vi "RotateToAngle.vi"(7 "X":dbl, 9 "Y":dbl, 11 "Z":dbl) -> ()   [LabVIEW 2017]
uses:
  <vilib>/Rock Robotics/WPI/ThirdParty/Phoenix-LabVIEW/Motor Controller/Controls/CTRE_Phoenix_MotorControl_ControlMode.ctl
  <vilib>/addons/control/pid/pid.llb/PID (DBL).vi
  <vilib>/addons/control/pid/NI_PID_pid.lvlib
panel:
  in  "Yaw":dbl
  in  "Rot. Point Y":dbl
  in  "Rot. Point X":dbl
  in  "Inputs":dbl[](array[numeric])
  out "Speed":dbl
  out "PID Values":cluster{"P":dbl, "I":dbl, "D":dbl}
  out "Motor Output":dbl
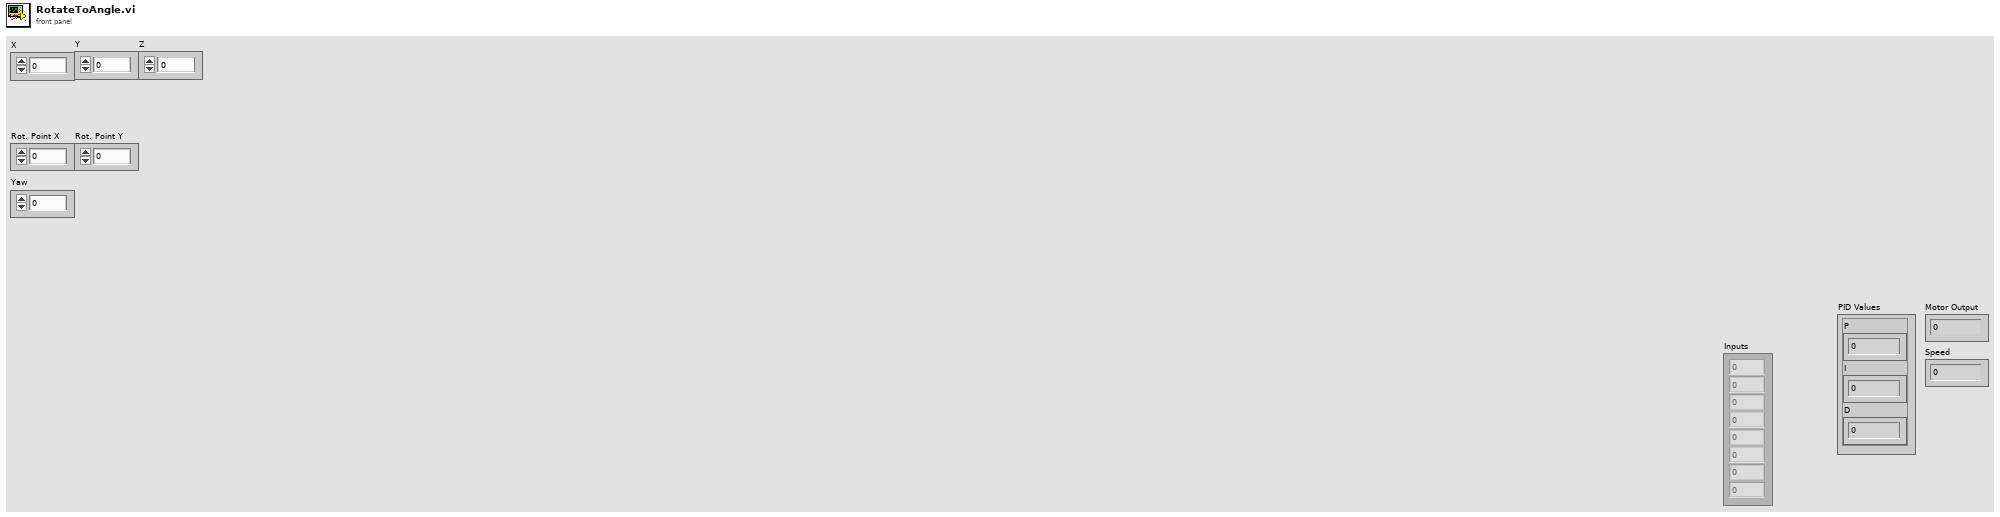
[diagram p1: front panel]
types:
  T1 = cluster{"proportional gain (Kc)":dbl, "integral time (Ti, min)":dbl, "derivative time (Td, min)":dbl}
  T2 = enum16{"Z Axis", "Y", "X", "Rot. Point X", "Rot. Point Y", "Width/2", "Max", "Length/2"}
  T3 = typedef "CTRE_Phoenix_MotorControl_ControlMode.ctl" = u16
  T4 = enum16{"Z", "Y", "X", "Rot. Point X", "Rot. Point Y", "Width/2", "Max", "Length/2"}
  T5 = typedef "WPI_AnalogChannelDevRef.ctl" = cluster{"DevStatus":errorcluster, "Analog Channel":T6}
  T6 = typedef "FPGA_AIChannel.ctl" = enum8{"AI 0", "AI 1", "AI 2", "AI 3", "AI MXP 0", "AI MXP 1", "AI MXP 2", "AI MXP 3", "Invalid"}
  T7 = typedef "WPI_MotorControlDeviceRef.ctl" = cluster{"DeviceStatus":errorcluster, "Type":T8, "PWM":cluster{"PWM Channel":T9, "DeadBand":T10}, "CAN":cluster{"Device Number":u8, "SetOutput VI Ref":variant, "GetOutput VI Ref":variant, "Enable VI Ref":variant, "Disable VI Ref":variant, "Data":variant}, "Invert":bool, "DIO PWM":cluster{"PWM \"Enable\" Channel":T9, "DIOChannel":T11, "PWM Rate":dbl}}
  T8 = typedef "WPI_MotorControlType.ctl" = enum16{"PWM", "CAN", "DIO PWM"}
  T9 = typedef "FPGA_DIOPWMChannel.ctl" = enum8{"PWM 0", "PWM 1", "PWM 2", "PWM 3", "PWM 4", "PWM 5", "PWM 6", "PWM 7", "PWM 8", "PWM 9", "PWM MXP 0", "PWM MXP 1", "PWM MXP 2", "PWM MXP 3", "PWM MXP 4", "PWM MXP 5", "PWM MXP 6", "PWM MXP 7", "PWM MXP 8", "PWM MXP 9", "Invalid"}
  T10 = typedef "WPI_PWMDeadband.ctl" = cluster{"Name":string, "maxPositivePwm":i32, "minPositivePwm":i32, "centerPwm":i32, "maxNegativePwm":i32, "minNegativePwm":i32, "angularRange":u16}
  T11 = typedef "FPGA_DIOChannel.ctl" = enum8{"DIO 0", "DIO 1", "DIO 2", "DIO 3", "DIO 4", "DIO 5", "DIO 6", "DIO 7", "DIO 8", "DIO 9", "DIO MXP 0", "DIO MXP 1", "DIO MXP 2", "DIO MXP 3", "DIO MXP 4", "DIO MXP 5", "DIO MXP 6", "DIO MXP 7", "DIO MXP 8", "DIO MXP 9", "DIO MXP 10", "DIO MXP 11", "DIO MXP 12", "DIO MXP 13", "DIO MXP 14", "DIO MXP 15", "SPI Port CS1", "SPI Port CS2", "SPI Port CS3", "SPI Port MISO", "SPI Port MOSI", "Invalid"}
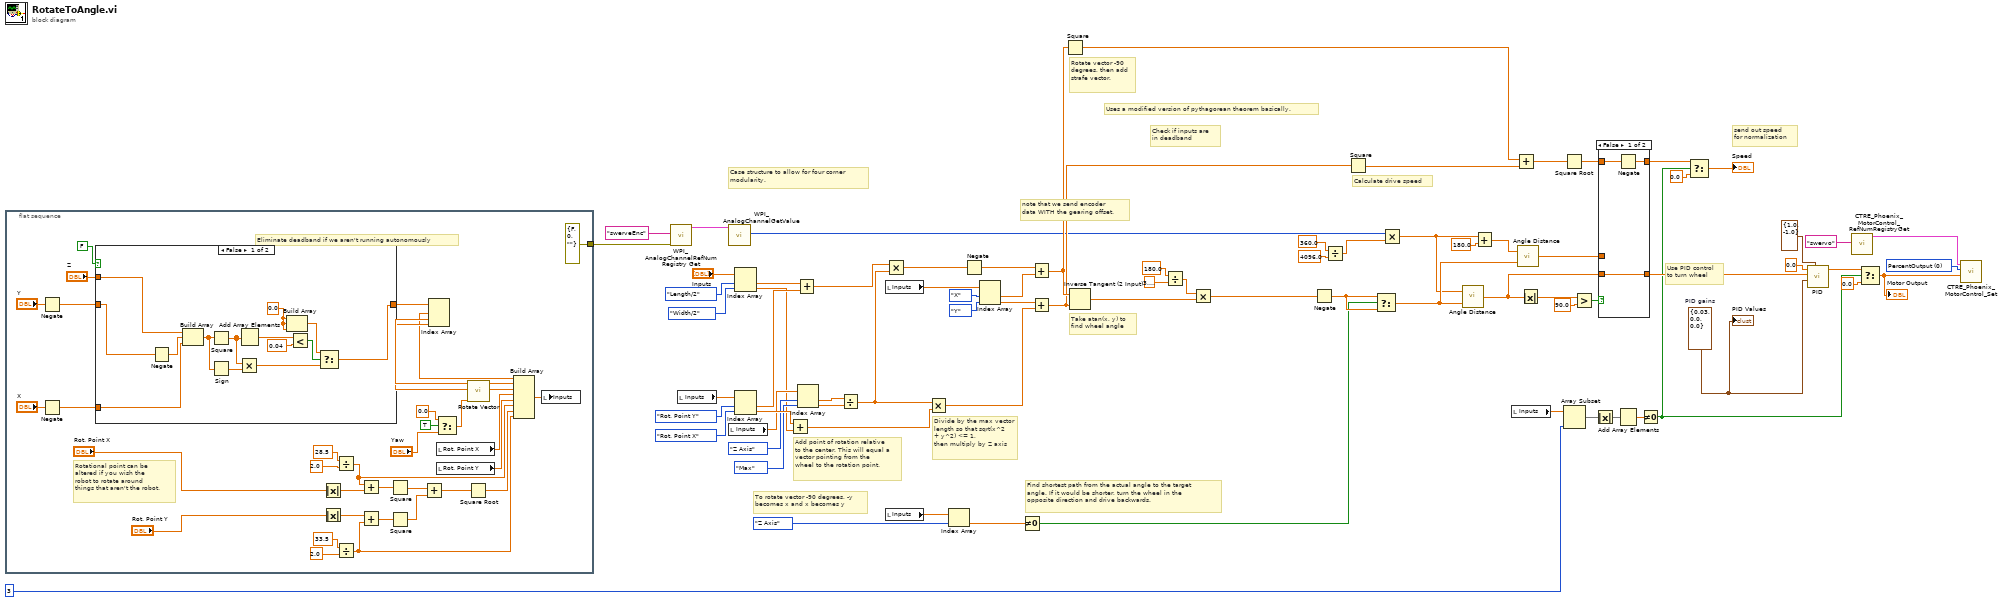
[diagram p0: block diagram]
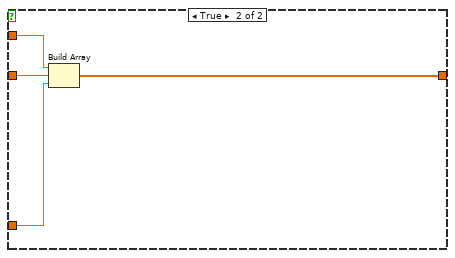
[diagram p2: hidden frame]
diagram:
  w75 = T1 {"proportional gain (Kc)"=0.03, "integral time (Ti, min)"=0.0, "derivative time (Td, min)"=0.0}  # PID gains
  w57 = T3 0 items=["PercentOutput"=0, "Position"=1, "Velocity"=2, "Current"=3, "Follower"=5, "MotionProfile"=6, "MotionMagic"=7, "MotionMagicArc"=8, "MotionProfileArc"=10, "Disabled"=15] ("Control Mode")
  # "Uses a modified version of pythagorean theorem basically."
  # "note that we send encoder \ndata WITH the gearing offset."
  # "Case structure to allow for four corner\nmodularity."
  # "To rotate vector -90 degrees, -y becomes x and x becomes y"
  # "send out speed\nfor normalization"
  # "Use PID control\nto turn wheel"
  # "Find shortest path from the actual angle to the target angle. If it would be shorter, turn the wheel in the opposite direction and drive backwards."
  # "Divide by the max vector length so that sqrt(x^2 + y^2) <= 1,\nthen multiply by Z axis"
  # "Add point of rotation relative to the center. This will equal a vector pointing from the\nwheel to the rotation point."
  # "Check if inputs are\nin deadband"
  # "Take atan(x, y) to find wheel angle"
  # "Calculate drive speed"
  # "Rotate vector -90 degrees, then add strafe vector."
  n1 = flat-sequence {
    tunnel: [errorcluster {"status"=FALSE, "code"=0, "source"=""} ("error constant")] -> w2
    frame #0 {
      # "Rotational point can be \naltered if you wish the \nrobot to rotate around \nthings that aren't the robot."
      # "Eliminate deadband if we aren't running autonomously"
      n2 = Negate(x="Y") -> (-x=w85:dbl)
      n3 = Negate(x="X") -> (-x=w84:dbl)
      n4 = case shown="False" FALSE {
        tunnel: w85 -> [w115 w128]
        tunnel: [w117 w129] -> w112
        tunnel: "Z" -> [w116 w131]
        tunnel: w84 -> [w114 w130]
        frame False {
          w123 = 0.0 ("element")
          n5 = Negate(x=w115) -> (-x=w119:dbl)
          n6 = Build Array(w116, w119, w114) -> (w122:dbl[])
          n7 = Square(x=w122) -> (x^2=w120:dbl[])
          n8 = Sign(1:w122) -> (0:w121:dbl[])
          n9 = Multiply(x=w120, y=w121) -> (x*y=w118:dbl[])
          n10 = Add Array Elements(numeric array=w120) -> (sum=w127:dbl)
          n11 = Build Array(w123, w123, w123) -> (w124:dbl[])
          n12 = Less?(x=w127, y=0.04 ("x")) -> (x < y?=w125:bool)
          n13 = Select(t=w124, s=w125, f=w118) -> (s? t:f=w117:dbl[])
        }
        frame True {
          n14 = Build Array(w131, w128, w130) -> (w129:dbl[])
        }
      }
      n15 = Absolute Value(x="Rot. Point X") -> (abs(x)=w101:dbl)
      n16 = Absolute Value(x="Rot. Point Y") -> (abs(x)=w98:dbl)
      n17 = Divide(x=28.5, y=2.0) -> (x/y=w89:dbl)
      n18 = Divide(x=33.5, y=2.0) -> (x/y=w87:dbl)
      n19 = Add(x=w89, y=w101) -> (x+y=w100:dbl)
      n20 = Add(x=w98, y=w87) -> (x+y=w99:dbl)
      n21 = Square(x=w100) -> (x^2=w96:dbl)
      n22 = Square(x=w99) -> (x^2=w97:dbl)
      n23 = Add(x=w96, y=w97) -> (x+y=w95:dbl)
      n24 = Index Array(array=w112) -> (element #1=w94:dbl, element #2=w108:dbl, element #3=w107:dbl)  [unwired: 3 in]
      n25 = local read "Rot. Point X"() -> (w91:dbl)
      n26 = local read "Rot. Point Y"() -> (w90:dbl)
      n27 = Select(t=0.0, s=TRUE, f="Yaw") -> (s? t:f=w106:dbl)
      n28 = call "Rotate Vector.vi"("Angle"=w106, "X"=w107, "Y"=w108) -> ("X'"=w92:dbl, "Y'"=w93:dbl)  [unwired: 7 in]
      n29 = Square Root(x=w95) -> (sqrt(x)=w88:dbl)
      n30 = Build Array(w94, w93, w92, w91, w90, w89, w88, w87) -> (w83:dbl[])
      n31 = local write "Inputs"(w83) -> ()
    }
  }
  n32 = call <vilib>:"WPI_AnalogChannelRefNum Registry Get.vi"("error in (no error)"=w2, "refnum name"="swerveEnc") -> ("AIDeviceRef"=w4:T5)  [unwired: 8 in, 1 out]
  n33 = local read "Inputs"() -> (w37:dbl[])
  n34 = call <vilib>:"WPI_AnalogChannelGetValue.vi"("AIDeviceRef"=w4) -> ("Value"=w9:i16)  [unwired: 8 in, 2 out]
  n35 = local read "Inputs"() -> (w34:dbl[])
  n36 = Index Array(array="Inputs", index #1=T4."Length/2", index #2=T4."Width/2") -> (element #1=w11:dbl, element #2=w10:dbl)
  n37 = Index Array(array=w37, index #1=T4."Rot. Point Y", index #2=T4."Rot. Point X") -> (element #1=w39:dbl, element #2=w38:dbl)
  n38 = Add(x=w38, y=w10) -> (x+y=w25:dbl)
  n39 = Add(x=w11, y=w39) -> (x+y=w40:dbl)
  n40 = Index Array(array=w34, index #1=T2."Z Axis", index #2=T4."Max") -> (element #1=w55:dbl, element #2=w56:dbl)
  n41 = Divide(x=w55, y=w56) -> (x/y=w67:dbl)
  n42 = Multiply(x=w40, y=w67) -> (x*y=w32:dbl)
  n43 = local read "Inputs"() -> (w52:dbl[])
  n44 = local read "Inputs"() -> (w69:dbl[])
  n45 = Multiply(x=w67, y=w25) -> (x*y=w29:dbl)
  n46 = Index Array(array=w69, index=T2."Z Axis") -> (element=w71:dbl)
  n47 = Negate(x=w32) -> (-x=w33:dbl)
  n48 = Index Array(array=w52, index #1=T4."X", index #2=T4."Y") -> (element #1=w53:dbl, element #2=w54:dbl)
  n49 = Not Equal To 0?(x=w71) -> (x != 0?=w72:bool)
  n50 = Add(x=w33, y=w53) -> (x+y=w31:dbl)
  n51 = Add(x=w54, y=w29) -> (x+y=w30:dbl)
  n52 = Square(x=w31) -> (x^2=w28:dbl)
  n53 = Inverse Tangent (2 Input)(1:w30, 2:w31) -> (0:w18:dbl)
  n54 = Divide(x=180.0 ("y"), y=3.141592653589793) -> (x/y=w21:dbl)
  n55 = Multiply(x=w21, y=w18) -> (x*y=w73:dbl)
  n56 = Negate(x=w73) -> (-x=w74:dbl)
  n57 = Divide(x=360.0, y=4096.0) -> (x/y=w5:dbl)
  n58 = Square(x=w30) -> (x^2=w19:dbl)
  n59 = Select(t=w74, s=w72, f=w74) -> (s? t:f=w68:dbl)
  n60 = Multiply(x=w9, y=w5) -> (x*y=w8:dbl)
  n61 = call "Angle Distance.vi"("Target Angle"=w68, "Current Angle"=w8) -> ("Distance"=w64:dbl)
  n62 = Add(x=w8, y=180.0) -> (x+y=w59:dbl)
  n63 = local read "Inputs"() -> (w45:dbl[])
  n64 = Add(x=w28, y=w19) -> (x+y=w20:dbl)
  n65 = call "Angle Distance.vi"("Target Angle"=w68, "Current Angle"=w59) -> ("Distance"=w60:dbl)
  n66 = Absolute Value(x=w64) -> (abs(x)=w65:dbl)
  n67 = Square Root(x=w20) -> (sqrt(x)=w61:dbl)
  n68 = Array Subset(array=w45, length=3) -> (w43:dbl[])  [unwired: 1 in]
  n69 = Greater?(x=w65, y=90.0) -> (0:w63:bool)
  n70 = Absolute Value(x=w43) -> (abs(x)=w44:dbl[])
  n71 = case shown="False" w63 {
    tunnel: w61 -> [w133 w135]
    tunnel: w64 -> [w134 _]
    tunnel: w60 -> [_ w136]
    tunnel: [w132 w135] -> w62
    tunnel: [w134 w136] -> w77
    frame False {
      n72 = Negate(x=w133) -> (-x=w132:dbl)
    }
    frame True {
    }
  }
  n73 = Add Array Elements(numeric array=w44) -> (sum=w42:dbl)
  n74 = Not Equal To 0?(x=w42) -> (x != 0?=w51:bool)
  n75 = Select(t=w62, s=w51, f=0.0) -> (s? t:f=→"Speed":dbl)
  n76 = call-poly <vilib>:"PID.vi"("output range"=cluster{"output high":dbl, "output low":dbl} {"output high"=1.0, "output low"=-1.0}, "PID gains"=w75, "process variable"=w77, "setpoint"=0.0) -> ("output"=w49:dbl)  [unwired: 6 in, 1 out]
  n77 = call <vilib>:"CTRE_Phoenix_MotorControl_RefNumRegistryGet.vi"("refnum name"="swervo") -> ("PhoenixMotorControlDevRef"=w14:T7)  [unwired: 9 in, 1 out]
  n78 = Select(t=w49, s=w51, f=0.0) -> (s? t:f=w12:dbl)
  "Motor Output" <- w12
  n79 = call <vilib>:"CTRE_Phoenix_MotorControl_Set.vi"("Output"=w12, "Control Mode"=w57, "PhoenixMotorControlDevRef"=w14) -> ()  [unwired: 7 in, 2 out]
  "PID Values" <- w75
